vi "Translator.Translate.Event.vi"   [LabVIEW 2019, in "Tools.lvlib"]
uses:
  Tools.lvlib
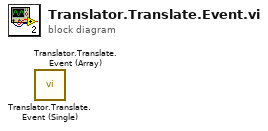
[diagram p0: block diagram]
diagram:
  n1 = call "Translator.Translate.Event (Single).vi"() -> ()  [unwired: 10 in, 2 out]
  n2 = call "Translator.Translate.Event (Array).vi"() -> ()  [unwired: 10 in, 2 out]
